vi "Motorcontroller Mode Set and Channel commands.vi"() -> ()   [LabVIEW 2009]
uses:
  <vilib>/Instr/_visa.llb/VISA Configure Serial Port (Instr).vi
panel:
  out "Heartbeat":bool
  out "All Stop":bool
  out "Set Mode 3":bool
  in  "Mode command 3":string="^04 C0"
  out "Set Mode 2":bool
  in  "Mode command 2":string="^03 00"
  in  "Mode command 1":string="^01 C4"
  out "Set RS232 Control":bool
  out "Set Mode 1":bool
  in  "Stop":bool
  in  "Turn Radius":i32=1
  in  "Turn Speed":i32=1
  in  "VISA resource name":refnum<visa-resource-name>="COM3"
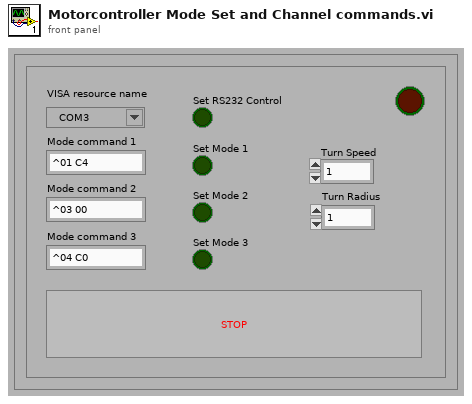
[diagram p1: front panel]
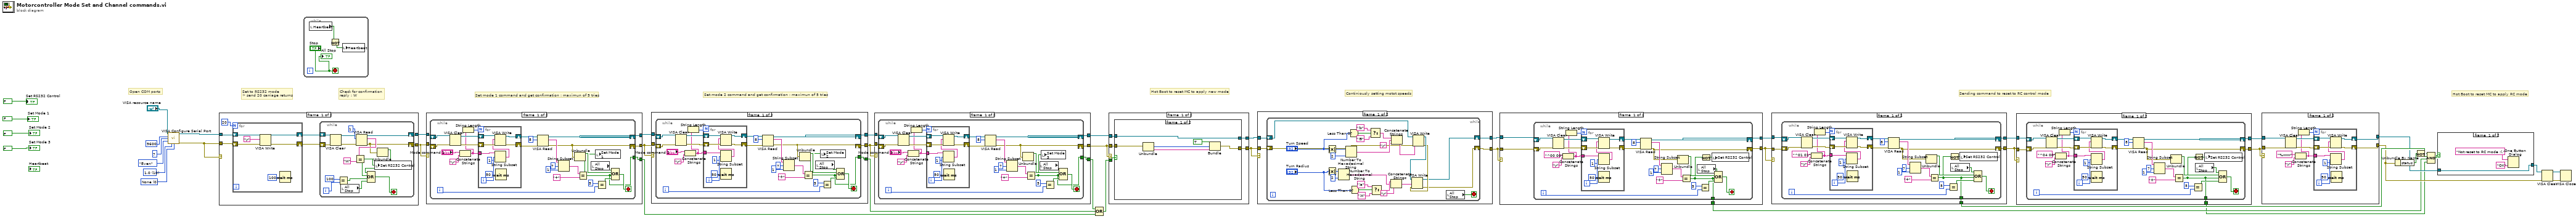
[diagram p0: block diagram]
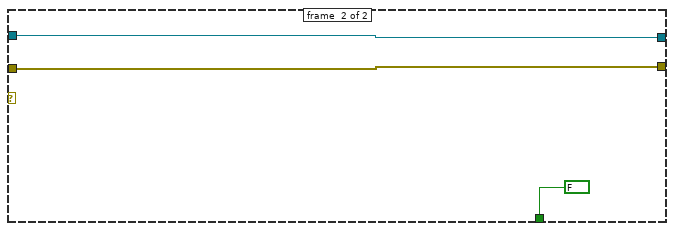
[diagram p2: hidden frame]
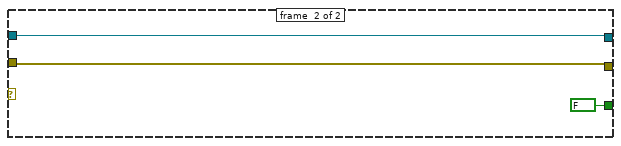
[diagram p3: hidden frame]
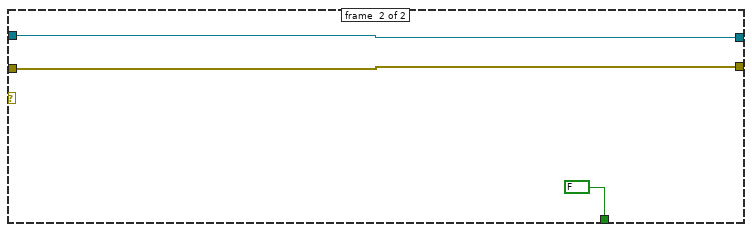
[diagram p4: hidden frame]
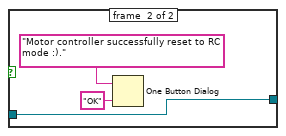
[diagram p6: hidden frame]
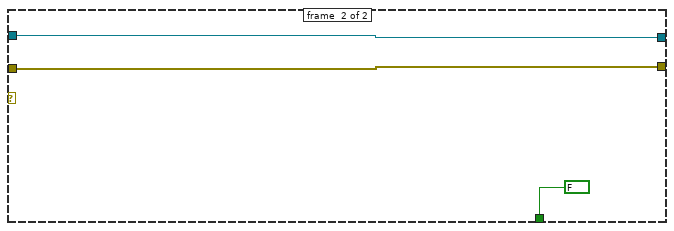
[diagram p7: hidden frame]
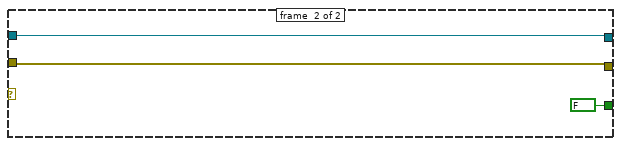
[diagram p8: hidden frame]
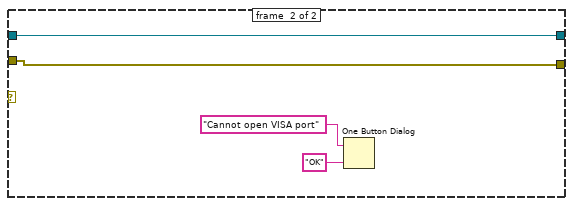
[diagram p10: hidden frame]
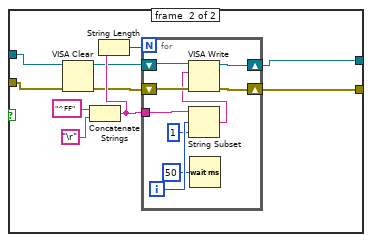
[diagram p11: hidden frame]
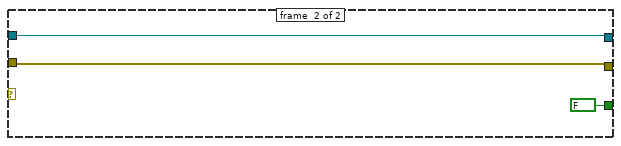
[diagram p13: hidden frame]
diagram:
  w40 = u16 0 items=["None", "XON/XOFF", "RTS/CTS", "XON/XOFF & RTS/CTS", "DTR/DSR", "XON/XOFF & DTR/DSR"] ("flow control (0:none)")
  w41 = u16 10 items=["1.0"=10, "1.5"=15, "2.0"=20] ("stop bits (10: 1 bit)")
  # "Continiously setting motot speeds"
  # "Sending command to reset to RC control mode"
  # "Set mode 2 command and get confirmation : maximun of 5 tries"
  # "Hot Boot to reset MC to apply RC mode"
  # "Hot Boot to reset MC to apply new mode"
  # "Check for confirmation\nreply : W"
  # "Set mode 1 command and get confirmation : maximun of 5 tries"
  # "Set to RS232 mode\n> send 20 carriage returns"
  # "Open COM ports"
  n1 = call-poly "VISA Configure Serial Port"("VISA resource name"="VISA resource name", "baud rate (9600)"=u32 9600, "data bits (8)"=u16 7, "parity (0:none)"=enum16{"None", "Odd", "Even", "Mark", "Space"}."Even", "stop bits (10: 1 bit)"=w41, "flow control (0:none)"=w40) -> ("VISA resource name out"=w39:refnum<visa-resource-name>, "error out"=w35:errorcluster)  [unwired: 1 in, 7 out]
  n2 = case shown="No Error" w35 {
    tunnel: w35 -> [w51 w77]
    tunnel: w39 -> [w50 w78]
    tunnel: [w49 w78] -> w38
    tunnel: [w46 w77] -> w36
    frame #0 {
      n3 = for {
        N: 20 -> [_]
        shift-right: [w71] -> w48
        shift-left: w51 -> [w74]
        shift-right: [w73] -> w47
        shift-left: w50 -> [w72]
        n4 = VISA Write(VISA resource name=w72, write buffer="\r", error in (no error)=w74) -> (VISA resource name out=w73:refnum<visa-resource-name>, error out=w71:errorcluster)  [unwired: 1 out]
        n5 = Wait (ms)(milliseconds to wait=u32 100) -> ()  [unwired: 1 out]
      }
      n6 = while {
        shift-right: [w64] -> w49
        shift-left: w47 -> [w65]
        shift-right: [w56] -> w46
        shift-left: w48 -> [w63]
        i -> [w60]
        stop <- w57 stop-if-true
        n7 = VISA Clear(VISA resource name=w65, error in (no error)=w63) -> (VISA resource name out=w62:refnum<visa-resource-name>, error out=w55:errorcluster)
        n8 = Equal?(x=100, y=w60) -> (x = y?=w58:bool)
        n9 = local read "All Stop"() -> (w53:bool)
        n10 = VISA Read(VISA resource name=w62, byte count=u32 1, error in (no error)=w55) -> (VISA resource name out=w64:refnum<visa-resource-name>, read buffer=w67:string, error out=w56:errorcluster)  [unwired: 1 out]
        n11 = Equal?(x=w67, y="W") -> (x = y?=w54:bool)
        n12 = local write "Set RS232 Control"(w54) -> ()
        n13 = Unbundle(w56) -> ("status"=w61:bool)  [unwired: 2 out]
        n14 = Compound Arithmetic op=OR(w61, w54, w58, w53) -> (w57:bool)
      }
    }
    frame #1 {
      n15 = One Button Dialog(message="Cannot open VISA port", button name ("OK")="OK") -> ()  [unwired: 1 out]
    }
  }
  n16 = while {
    stop <- "Stop" stop-if-true
    n17 = local read "Heartbeat"() -> (w80:bool)
    n18 = Not(x=w80) -> (.not. x?=w79:bool)
    n19 = local write "Heartbeat"(w79) -> ()
    "All Stop" <- "Stop"
  }
  n20 = case shown="No Error" w36 {
    tunnel: [w86 w123] -> w28
    tunnel: [w85 w122] -> w29
    tunnel: w38 -> [w84 w123]
    tunnel: w36 -> [w83 w122]
    tunnel: [w82 FALSE] -> w30
    frame #0 {
      n21 = while {
        shift-right: [w107] -> w86
        shift-left: w84 -> [w111]
        shift-right: [w94] -> w85
        shift-left: w83 -> [w110]
        tunnel: [w88] -> w82
        i -> [w91]
        stop <- w89 stop-if-true
        n22 = VISA Clear(VISA resource name=w111, error in (no error)=w110) -> (VISA resource name out=w104:refnum<visa-resource-name>, error out=w103:errorcluster)
        n23 = Concatenate Strings("Mode command 1", "\r") -> (w95:string)
        n24 = String Length(string=w95) -> (length=w96:i32)
        n25 = for {
          N: w96 -> [_]
          tunnel: w95 -> [w116]
          shift-right: [w120] -> w109
          shift-left: w103 -> [w117]
          shift-right: [w119] -> w108
          shift-left: w104 -> [w118]
          i -> [w115]
          n26 = String Subset(string=w116, offset (0)=w115, length (rest)=1 ("length (rest)")) -> (substring=w113:string)
          n27 = VISA Write(VISA resource name=w118, write buffer=w113, error in (no error)=w117) -> (VISA resource name out=w119:refnum<visa-resource-name>, error out=w120:errorcluster)  [unwired: 1 out]
          n28 = Wait (ms)(milliseconds to wait=u32 50) -> ()  [unwired: 1 out]
        }
        n29 = VISA Read(VISA resource name=w108, byte count=u32 8, error in (no error)=w109) -> (VISA resource name out=w107:refnum<visa-resource-name>, read buffer=w100:string, error out=w94:errorcluster)  [unwired: 1 out]
        n30 = String Subset(string=w100, offset (0)=7, length (rest)=1 ("length (rest)")) -> (substring=w99:string)
        n31 = Unbundle(w94) -> ("status"=w90:bool)  [unwired: 2 out]
        n32 = Equal?(x=w99, y="+") -> (x = y?=w88:bool)
        n33 = local read "All Stop"() -> (w87:bool)
        n34 = local write "Set Mode 1"(w88) -> ()
        n35 = Equal?(x=5, y=w91) -> (x = y?=w92:bool)
        n36 = Compound Arithmetic op=OR(w87, w90, w88, w92) -> (w89:bool)
      }
    }
    frame #1 {
    }
  }
  n37 = case shown="No Error" w29 {
    tunnel: [w128 w165] -> w15
    tunnel: [w127 w164] -> w14
    tunnel: w28 -> [w126 w165]
    tunnel: w29 -> [w125 w164]
    tunnel: [w124 FALSE] -> w16
    frame #0 {
      n38 = while {
        shift-right: [w149] -> w128
        shift-left: w126 -> [w153]
        shift-right: [w136] -> w127
        shift-left: w125 -> [w152]
        tunnel: [w130] -> w124
        i -> [w133]
        stop <- w131 stop-if-true
        n39 = VISA Clear(VISA resource name=w153, error in (no error)=w152) -> (VISA resource name out=w146:refnum<visa-resource-name>, error out=w145:errorcluster)
        n40 = Concatenate Strings("Mode command 2", "\r") -> (w137:string)
        n41 = String Length(string=w137) -> (length=w138:i32)
        n42 = for {
          N: w138 -> [_]
          tunnel: w137 -> [w158]
          shift-right: [w162] -> w151
          shift-left: w145 -> [w159]
          shift-right: [w161] -> w150
          shift-left: w146 -> [w160]
          i -> [w157]
          n43 = String Subset(string=w158, offset (0)=w157, length (rest)=1 ("length (rest)")) -> (substring=w155:string)
          n44 = VISA Write(VISA resource name=w160, write buffer=w155, error in (no error)=w159) -> (VISA resource name out=w161:refnum<visa-resource-name>, error out=w162:errorcluster)  [unwired: 1 out]
          n45 = Wait (ms)(milliseconds to wait=u32 50) -> ()  [unwired: 1 out]
        }
        n46 = VISA Read(VISA resource name=w150, byte count=u32 8, error in (no error)=w151) -> (VISA resource name out=w149:refnum<visa-resource-name>, read buffer=w142:string, error out=w136:errorcluster)  [unwired: 1 out]
        n47 = String Subset(string=w142, offset (0)=7, length (rest)=1 ("length (rest)")) -> (substring=w141:string)
        n48 = Unbundle(w136) -> ("status"=w132:bool)  [unwired: 2 out]
        n49 = Equal?(x=w141, y="+") -> (x = y?=w130:bool)
        n50 = local read "All Stop"() -> (w129:bool)
        n51 = local write "Set Mode 2"(w130) -> ()
        n52 = Equal?(x=5, y=w133) -> (x = y?=w134:bool)
        n53 = Compound Arithmetic op=OR(w129, w132, w130, w134) -> (w131:bool)
      }
    }
    frame #1 {
    }
  }
  n54 = case shown="No Error" w14 {
    tunnel: [w170 w207] -> w12
    tunnel: [w169 w206] -> w1
    tunnel: w15 -> [w168 w207]
    tunnel: w14 -> [w167 w206]
    tunnel: [w166 FALSE] -> w11
    frame #0 {
      n55 = while {
        shift-right: [w191] -> w170
        shift-left: w168 -> [w195]
        shift-right: [w178] -> w169
        shift-left: w167 -> [w194]
        tunnel: [w172] -> w166
        i -> [w175]
        stop <- w173 stop-if-true
        n56 = VISA Clear(VISA resource name=w195, error in (no error)=w194) -> (VISA resource name out=w188:refnum<visa-resource-name>, error out=w187:errorcluster)
        n57 = Concatenate Strings("Mode command 3", "\r") -> (w179:string)
        n58 = String Length(string=w179) -> (length=w180:i32)
        n59 = for {
          N: w180 -> [_]
          tunnel: w179 -> [w200]
          shift-right: [w204] -> w193
          shift-left: w187 -> [w201]
          shift-right: [w203] -> w192
          shift-left: w188 -> [w202]
          i -> [w199]
          n60 = String Subset(string=w200, offset (0)=w199, length (rest)=1 ("length (rest)")) -> (substring=w197:string)
          n61 = VISA Write(VISA resource name=w202, write buffer=w197, error in (no error)=w201) -> (VISA resource name out=w203:refnum<visa-resource-name>, error out=w204:errorcluster)  [unwired: 1 out]
          n62 = Wait (ms)(milliseconds to wait=u32 50) -> ()  [unwired: 1 out]
        }
        n63 = VISA Read(VISA resource name=w192, byte count=u32 8, error in (no error)=w193) -> (VISA resource name out=w191:refnum<visa-resource-name>, read buffer=w184:string, error out=w178:errorcluster)  [unwired: 1 out]
        n64 = String Subset(string=w184, offset (0)=7, length (rest)=1 ("length (rest)")) -> (substring=w183:string)
        n65 = Unbundle(w178) -> ("status"=w174:bool)  [unwired: 2 out]
        n66 = Equal?(x=w183, y="+") -> (x = y?=w172:bool)
        n67 = local read "All Stop"() -> (w171:bool)
        n68 = local write "Set Mode 3"(w172) -> ()
        n69 = Equal?(x=5, y=w175) -> (x = y?=w176:bool)
        n70 = Compound Arithmetic op=OR(w171, w174, w172, w176) -> (w173:bool)
      }
    }
    frame #1 {
    }
  }
  n71 = Compound Arithmetic op=OR(w11, w16, w30) -> (w31:bool)
  n72 = case shown="No Error" w1 {
    tunnel: w1 -> [w212 w239]
    tunnel: w12 -> [w211 w238]
    tunnel: w31 -> [w208 _]
    tunnel: [w210 w239] -> w34
    tunnel: [w209 w238] -> w45
    frame #0 {
      n73 = case shown="True" w208 {
        tunnel: w212 -> [w217 w222]
        tunnel: w211 -> [w213 w221]
        tunnel: [w218 w220] -> w210
        tunnel: [w213 w219] -> w209
        frame #0 {
          n74 = Unbundle(w217) -> ("code"=w215:i32, "source"=w216:string)  [unwired: 1 out]
          n75 = Bundle(TRUE, "code"=w215, "source"=w216) -> (w218:cluster{bool, "code":i32, "source":string})  [unwired: 1 out]
        }
        frame #1 {
          n76 = VISA Clear(VISA resource name=w221, error in (no error)=w222) -> (VISA resource name out=w225:refnum<visa-resource-name>, error out=w226:errorcluster)
          n77 = Concatenate Strings("^FF" ("string"), "\r") -> (w228:string)
          n78 = String Length(string=w228) -> (length=w227:i32)
          n79 = for {
            N: w227 -> [_]
            tunnel: w228 -> [w233]
            shift-right: [w237] -> w220
            shift-left: w226 -> [w234]
            shift-right: [w236] -> w219
            shift-left: w225 -> [w235]
            i -> [w232]
            n80 = String Subset(string=w233, offset (0)=w232, length (rest)=1 ("length (rest)")) -> (substring=w230:string)
            n81 = VISA Write(VISA resource name=w235, write buffer=w230, error in (no error)=w234) -> (VISA resource name out=w236:refnum<visa-resource-name>, error out=w237:errorcluster)  [unwired: 1 out]
            n82 = Wait (ms)(milliseconds to wait=u32 50) -> ()  [unwired: 1 out]
          }
        }
      }
    }
    frame #1 {
    }
  }
  n83 = case shown="No Error" w34 {
    tunnel: w34 -> [w243 w271]
    tunnel: [w242 w272] -> w20
    tunnel: [w241 w271] -> w19
    tunnel: w45 -> [w240 w272]
    frame #0 {
      n84 = while {
        shift-right: [w248] -> w242
        shift-left: w240 -> [w253]
        shift-right: [w247] -> w241
        shift-left: w243 -> [w252]
        stop <- w244 stop-if-true
        n85 = Absolute Value(x="Turn Speed") -> (abs(x)=w270:i32)
        n86 = Absolute Value(x="Turn Radius") -> (abs(x)=w269:i32)
        n87 = Number To Hexadecimal String(1:i16 2 ("width (-)"), 2:w269) -> (0:w255:string)
        n88 = Number To Hexadecimal String(1:i16 2 ("width (-)"), 2:w270) -> (0:w257:string)
        n89 = Less Than 0?(x="Turn Speed") -> (x < 0?=w266:bool)
        n90 = Less Than 0?(x="Turn Radius") -> (x < 0?=w260:bool)
        n91 = Select(t="!b", s=w266, f="!B") -> (s? t:f=w258:string)
        n92 = Select(t="!a", s=w260, f="!A") -> (s? t:f=w256:string)
        n93 = Concatenate Strings(w256, w255, "\r") -> (w251:string)
        n94 = Concatenate Strings(w258, w257, "\r") -> (w254:string)
        n95 = VISA Write(VISA resource name=w253, write buffer=w254, error in (no error)=w252) -> (VISA resource name out=w250:refnum<visa-resource-name>, error out=w249:errorcluster)  [unwired: 1 out]
        n96 = VISA Write(VISA resource name=w250, write buffer=w251, error in (no error)=w249) -> (VISA resource name out=w248:refnum<visa-resource-name>, error out=w247:errorcluster)  [unwired: 1 out]
        n97 = local read "All Stop"() -> (w244:bool)
      }
    }
    frame #1 {
    }
  }
  n98 = case shown="No Error" w19 {
    tunnel: w20 -> [w277 w315]
    tunnel: [w276 w315] -> w18
    tunnel: w19 -> [w274 w314]
    tunnel: [w275 w314] -> w17
    tunnel: [w273 FALSE] -> w7
    frame #0 {
      n99 = while {
        shift-right: [w299] -> w276
        shift-left: w277 -> [w303]
        shift-right: [w282] -> w275
        shift-left: w274 -> [w302]
        tunnel: [w279] -> w273
        i -> [w285]
        stop <- w283 stop-if-true
        n100 = VISA Clear(VISA resource name=w303, error in (no error)=w302) -> (VISA resource name out=w297:refnum<visa-resource-name>, error out=w296:errorcluster)
        n101 = Concatenate Strings("^00 00" ("string"), "\r") -> (w288:string)
        n102 = String Length(string=w288) -> (length=w289:i32)
        n103 = for {
          N: w289 -> [_]
          tunnel: w288 -> [w308]
          shift-right: [w312] -> w301
          shift-left: w296 -> [w309]
          shift-right: [w311] -> w300
          shift-left: w297 -> [w310]
          i -> [w307]
          n104 = String Subset(string=w308, offset (0)=w307, length (rest)=1 ("length (rest)")) -> (substring=w305:string)
          n105 = VISA Write(VISA resource name=w310, write buffer=w305, error in (no error)=w309) -> (VISA resource name out=w311:refnum<visa-resource-name>, error out=w312:errorcluster)  [unwired: 1 out]
          n106 = Wait (ms)(milliseconds to wait=u32 50) -> ()  [unwired: 1 out]
        }
        n107 = VISA Read(VISA resource name=w300, byte count=u32 8, error in (no error)=w301) -> (VISA resource name out=w299:refnum<visa-resource-name>, read buffer=w293:string, error out=w282:errorcluster)  [unwired: 1 out]
        n108 = String Subset(string=w293, offset (0)=7, length (rest)=1 ("length (rest)")) -> (substring=w292:string)
        n109 = Unbundle(w282) -> ("status"=w284:bool)  [unwired: 2 out]
        n110 = Equal?(x=w292, y="+") -> (x = y?=w279:bool)
        n111 = local read "All Stop"() -> (w278:bool)
        n112 = Equal?(x=5, y=w285) -> (x = y?=w286:bool)
        n113 = Not(x=w279) -> (.not. x?=w280:bool)
        n114 = local write "Set RS232 Control"(w280) -> ()
        n115 = Compound Arithmetic op=OR(w278, w284, w279, w286) -> (w283:bool)
      }
    }
    frame #1 {
    }
  }
  n116 = case shown="No Error" w17 {
    tunnel: w18 -> [w320 w358]
    tunnel: [w319 w358] -> w6
    tunnel: w17 -> [w317 w357]
    tunnel: [w318 w357] -> w5
    tunnel: [w316 FALSE] -> w26
    frame #0 {
      n117 = while {
        shift-right: [w342] -> w319
        shift-left: w320 -> [w346]
        shift-right: [w326] -> w318
        shift-left: w317 -> [w345]
        tunnel: [w323] -> w316
        i -> [w328]
        stop <- w322 stop-if-true
        n118 = VISA Clear(VISA resource name=w346, error in (no error)=w345) -> (VISA resource name out=w340:refnum<visa-resource-name>, error out=w339:errorcluster)
        n119 = Concatenate Strings("^01 01" ("string"), "\r") -> (w331:string)
        n120 = String Length(string=w331) -> (length=w332:i32)
        n121 = for {
          N: w332 -> [_]
          tunnel: w331 -> [w351]
          shift-right: [w355] -> w344
          shift-left: w339 -> [w352]
          shift-right: [w354] -> w343
          shift-left: w340 -> [w353]
          i -> [w350]
          n122 = String Subset(string=w351, offset (0)=w350, length (rest)=1 ("length (rest)")) -> (substring=w348:string)
          n123 = VISA Write(VISA resource name=w353, write buffer=w348, error in (no error)=w352) -> (VISA resource name out=w354:refnum<visa-resource-name>, error out=w355:errorcluster)  [unwired: 1 out]
          n124 = Wait (ms)(milliseconds to wait=u32 50) -> ()  [unwired: 1 out]
        }
        n125 = VISA Read(VISA resource name=w343, byte count=u32 8, error in (no error)=w344) -> (VISA resource name out=w342:refnum<visa-resource-name>, read buffer=w336:string, error out=w326:errorcluster)  [unwired: 1 out]
        n126 = String Subset(string=w336, offset (0)=7, length (rest)=1 ("length (rest)")) -> (substring=w335:string)
        n127 = Unbundle(w326) -> ("status"=w327:bool)  [unwired: 2 out]
        n128 = Equal?(x=w335, y="+") -> (x = y?=w323:bool)
        n129 = Equal?(x=5, y=w328) -> (x = y?=w329:bool)
        n130 = Not(x=w323) -> (.not. x?=w324:bool)
        n131 = local read "All Stop"() -> (w321:bool)
        n132 = local write "Set RS232 Control"(w324) -> ()
        n133 = Compound Arithmetic op=OR(w321, w327, w323, w329) -> (w322:bool)
      }
    }
    frame #1 {
    }
  }
  n134 = case shown="No Error" w5 {
    tunnel: w6 -> [w363 w401]
    tunnel: [w362 w401] -> w4
    tunnel: w5 -> [w360 w400]
    tunnel: [w361 w400] -> w3
    tunnel: [w359 FALSE] -> w2
    frame #0 {
      n135 = while {
        shift-right: [w385] -> w362
        shift-left: w363 -> [w389]
        shift-right: [w369] -> w361
        shift-left: w360 -> [w388]
        tunnel: [w366] -> w359
        i -> [w371]
        stop <- w365 stop-if-true
        n136 = VISA Clear(VISA resource name=w389, error in (no error)=w388) -> (VISA resource name out=w383:refnum<visa-resource-name>, error out=w382:errorcluster)
        n137 = Concatenate Strings("^04 00" ("string"), "\r") -> (w374:string)
        n138 = String Length(string=w374) -> (length=w375:i32)
        n139 = for {
          N: w375 -> [_]
          tunnel: w374 -> [w394]
          shift-right: [w398] -> w387
          shift-left: w382 -> [w395]
          shift-right: [w397] -> w386
          shift-left: w383 -> [w396]
          i -> [w393]
          n140 = String Subset(string=w394, offset (0)=w393, length (rest)=1 ("length (rest)")) -> (substring=w391:string)
          n141 = VISA Write(VISA resource name=w396, write buffer=w391, error in (no error)=w395) -> (VISA resource name out=w397:refnum<visa-resource-name>, error out=w398:errorcluster)  [unwired: 1 out]
          n142 = Wait (ms)(milliseconds to wait=u32 50) -> ()  [unwired: 1 out]
        }
        n143 = VISA Read(VISA resource name=w386, byte count=u32 8, error in (no error)=w387) -> (VISA resource name out=w385:refnum<visa-resource-name>, read buffer=w379:string, error out=w369:errorcluster)  [unwired: 1 out]
        n144 = String Subset(string=w379, offset (0)=7, length (rest)=1 ("length (rest)")) -> (substring=w378:string)
        n145 = Unbundle(w369) -> ("status"=w370:bool)  [unwired: 2 out]
        n146 = Equal?(x=w378, y="+") -> (x = y?=w366:bool)
        n147 = Equal?(x=5, y=w371) -> (x = y?=w372:bool)
        n148 = Not(x=w366) -> (.not. x?=w367:bool)
        n149 = local read "All Stop"() -> (w364:bool)
        n150 = local write "Set RS232 Control"(w367) -> ()
        n151 = Compound Arithmetic op=OR(w364, w370, w366, w372) -> (w365:bool)
      }
    }
    frame #1 {
    }
  }
  n152 = case shown="No Error" w3 {
    tunnel: w4 -> [w411 w422]
    tunnel: w3 -> [w410 w421]
    tunnel: [w403 w422] -> w22
    tunnel: [w402 w421] -> w9
    frame #0 {
      n153 = VISA Clear(VISA resource name=w411, error in (no error)=w410) -> (VISA resource name out=w408:refnum<visa-resource-name>, error out=w407:errorcluster)
      n154 = Concatenate Strings("%rrrrrr" ("string"), "\r") -> (w405:string)
      n155 = String Length(string=w405) -> (length=w406:i32)
      n156 = for {
        N: w406 -> [_]
        tunnel: w405 -> [w416]
        shift-right: [w420] -> w402
        shift-left: w407 -> [w417]
        shift-right: [w419] -> w403
        shift-left: w408 -> [w418]
        i -> [w415]
        n157 = String Subset(string=w416, offset (0)=w415, length (rest)=1 ("length (rest)")) -> (substring=w413:string)
        n158 = VISA Write(VISA resource name=w418, write buffer=w413, error in (no error)=w417) -> (VISA resource name out=w419:refnum<visa-resource-name>, error out=w420:errorcluster)  [unwired: 1 out]
        n159 = Wait (ms)(milliseconds to wait=u32 50) -> ()  [unwired: 1 out]
      }
    }
    frame #1 {
    }
  }
  n160 = Unbundle By Name(w9) -> ("status"=w25:bool)
  n161 = Not(x=w25) -> (.not. x?=w21:bool)
  n162 = Compound Arithmetic op=AND(w21, w26, w7, w2) -> (w24:bool)
  n163 = case shown="True" w24 {
    tunnel: [w423 w426] -> w23
    tunnel: w22 -> [w423 w426]
    frame #0 {
      n164 = One Button Dialog(message="Not reset to RC mode :(.", button name ("OK")="OK") -> ()  [unwired: 1 out]
    }
    frame #1 {
      n165 = One Button Dialog(message="Motor controller successfully reset to RC mode :).", button name ("OK")="OK") -> ()  [unwired: 1 out]
    }
  }
  n166 = VISA Clear(VISA resource name=w23, error in (no error)=w9) -> (VISA resource name out=w10:refnum<visa-resource-name>, error out=w8:errorcluster)
  n167 = VISA Close(VISA resource name=w10, error in (no error)=w8) -> ()  [unwired: 1 out]
  "Set Mode 1" <- FALSE
  "Set RS232 Control" <- FALSE
  "Set Mode 2" <- FALSE
  "Set Mode 3" <- FALSE
